vi "WriteMotorCorrectionData.vi"(8 "error in (no error)":errorcluster, 10 "Motion Correction Data":dbl[](array[numeric]), 11 "AODAcq in":refnum<class "AODAcq.lvclass">) -> (0 "error out":errorcluster, 3 "AODAcq out":refnum<class "AODAcq.lvclass">)   [LabVIEW 2014, in "AODAcq.lvclass"]
uses:
  AODAcq.lvclass
  AODAcq.lvclass/AODAcq.ctl
  HDF5Tools/LabView/Append To Dataset 2D Double.vi
  HDF5Tools/LabView/HDF5Tools.lvlib
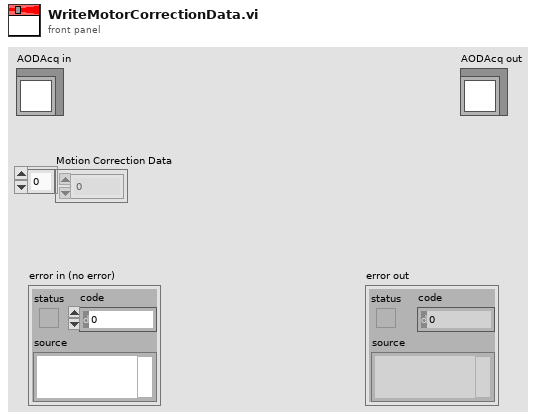
[diagram p1: front panel]
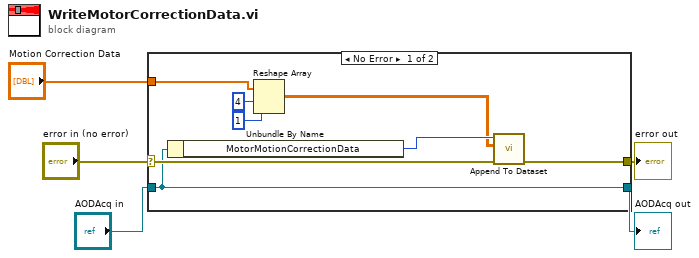
[diagram p0: block diagram]
diagram:
  n1 = case shown="No Error" "error in (no error)" {
    selector: "error in (no error)" -> [w12 w15]
    tunnel: [w11 w15] -> w4
    tunnel: [w10 w14] -> w2
    tunnel: "AODAcq in" -> [w10 w14]
    tunnel: "Motion Correction Data" -> [w9 _]
    frame No Error {
      n2 = Unbundle By Name(w10) -> ("MotorMotionCorrectionData"=w13:i32)
      n3 = Reshape Array(w9, 4 ("dimension size"), 1 ("dimension size")) -> (w6:dbl[][])
      n4 = call-poly "Append To Dataset.vi"("Error in (no error)"=w12, "Data"=w6, "Dataset id in"=w13) -> ("Error out"=w11:errorcluster)  [unwired: 7 in, 1 out]
    }
    frame Error {
    }
  }
  "error out" <- w4
  "AODAcq out" <- w2
